vi "Example_digital_out_speed_test.vi"() -> ()   [LabVIEW 2022 SP3]
uses:
  usbtmc_scpi_labtool.lvlib
panel:
  in  "stop":bool
  in  "VISA resource name in":refnum<visa-resource-name>="USB0::0xCAFE::0x4000::123456::INSTR"
  in  "Pin":u8 max=7 step=1
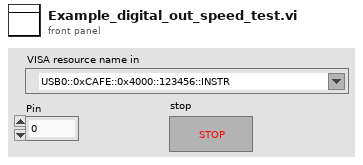
[diagram p1: front panel]
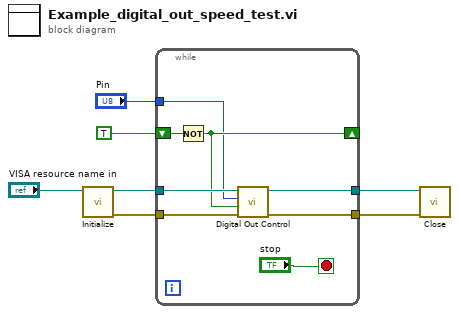
[diagram p0: block diagram]
diagram:
  n1 = call "Initialize.vi"("VISA resource name in"="VISA resource name in") -> ("error out"=w5:errorcluster, "VISA resource name out"=w7:refnum<visa-resource-name>)  [unwired: 9 in]
  n2 = while {
    tunnel: w7 -> [w13]
    tunnel: [w15] -> w6
    tunnel: w5 -> [w12]
    tunnel: [w14] -> w4
    tunnel: "Pin" -> [w9]
    shift-right: [w10] -> _
    shift-left: TRUE -> [w11]
    stop <- "stop" stop-if-true
    n3 = Not(x=w11) -> (.not. x?=w10:bool)
    n4 = call "Digital Out Control.vi"("VISA resource name"=w13, "Pin"=w9, "Enable Pin (F: Off)"=w10, "error in (no error)"=w12) -> ("VISA resource name out"=w15:refnum<visa-resource-name>, "error out"=w14:errorcluster)  [unwired: 5 in]
  }
  n5 = call "Close.vi"("error in (no error)"=w4, "VISA resource name"=w6) -> ()  [unwired: 10 in]
